vi "FRCts20_Backend_BinarySearchTeamNumber.vi"(8 "error in (no error)":errorcluster) -> (0 "error out":errorcluster)   [LabVIEW 2013, in "FRCts20_Backend_Engine_Deprecated.lvlib"]
doc: "Sorts all teams by team number and performs a binary search through the resulting array of teams. All it does is tell us if the team number was located."
uses:
  FRCts20_Backend_Engine_Deprecated.lvlib
  FRCts20_Backend_TeamDataDfn.ctl
  FRCts20_Backend_TeamDfn.ctl
  FRCts20_Backend_Team_Info.ctl
  FRCts20_Backend_IssueTeamList.ctl
  FRCts20_Backend_IssueDfn.ctl
  FRCts20_Backend_Note_list.ctl
  FRCts20_Backend_Note.ctl
  FRCts20_Backend_request_info.ctl
  FRCts20_Backend_Controls.lvlib
panel:
  out "Found?":bool
  in  "Team Number?":u16
  in  "TeamData":T1
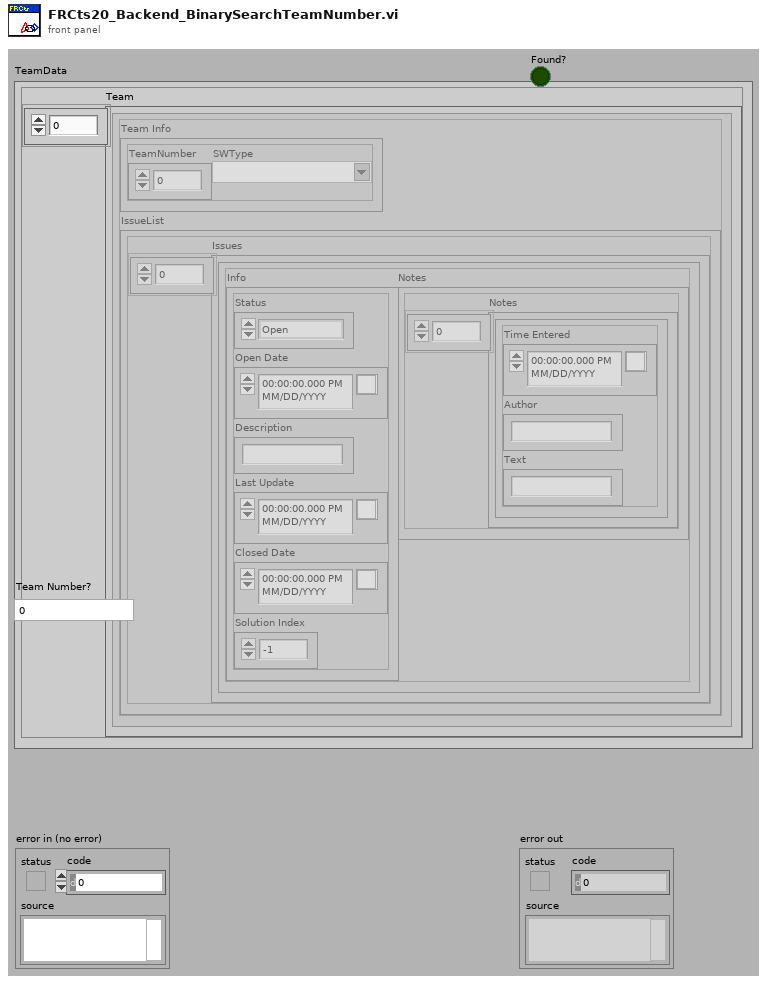
[diagram p1: front panel]
types:
  T1 = typedef "FRCts20_Backend_Controls.lvlib/FRCts20_Backend_TeamDataDfn.ctl" = cluster{"Team":T2[]}
  T2 = typedef "FRCts20_Backend_Controls.lvlib/FRCts20_Backend_TeamDfn.ctl" = cluster{"Team Info":T3, "IssueList":T4}
  T3 = typedef "FRCts20_Backend_Controls.lvlib/FRCts20_Backend_Team_Info.ctl" = cluster{"TeamNumber":u16, "SWType":string}
  T4 = typedef "FRCts20_Backend_Controls.lvlib/FRCts20_Backend_IssueTeamList.ctl" = cluster{"Issues":T5[]}
  T5 = typedef "FRCts20_Backend_Controls.lvlib/FRCts20_Backend_IssueDfn.ctl" = cluster{"Notes":T6, "Info":T8}
  T6 = typedef "FRCts20_Backend_Controls.lvlib/FRCts20_Backend_Note_list.ctl" = cluster{"Notes":T7[]}
  T7 = typedef "FRCts20_Backend_Controls.lvlib/FRCts20_Backend_Note.ctl" = cluster{"Time Entered":timestamp, "Author":string, "Text":string}
  T8 = typedef "FRCts20_Backend_Controls.lvlib/FRCts20_Backend_request_info.ctl" = cluster{"Status":enum16{"Open", "In Work", "Closed"}, "Open Date":timestamp, "Description":string, "Last Update":timestamp, "Closed Date":timestamp, "Solution Index":i32}
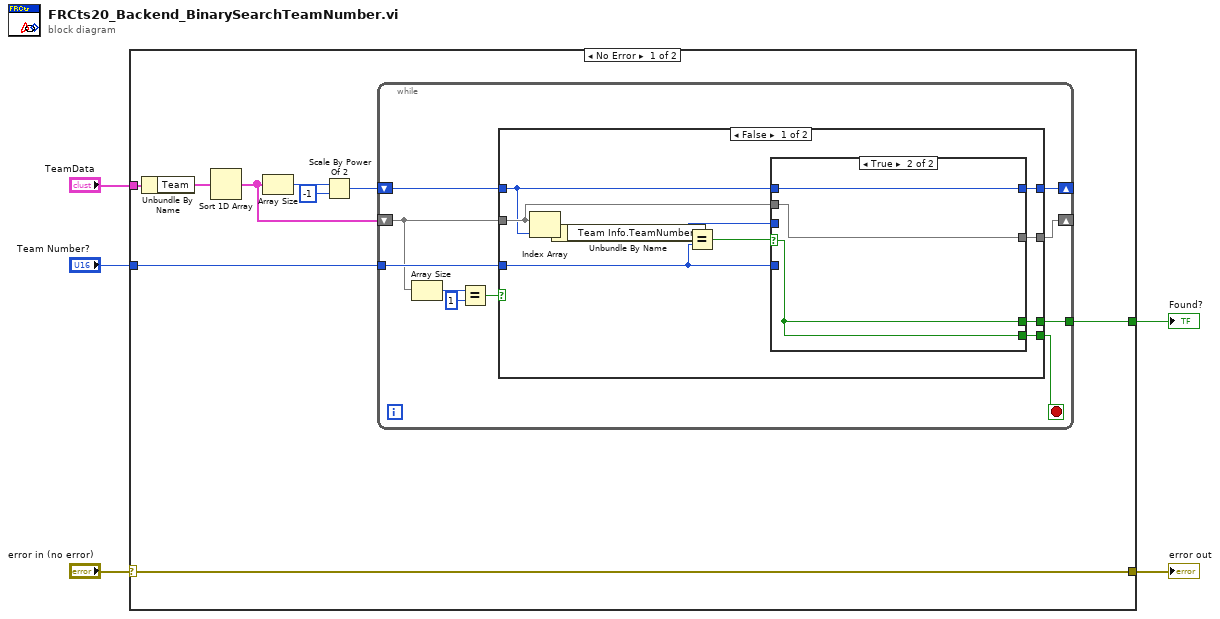
[diagram p0: block diagram]
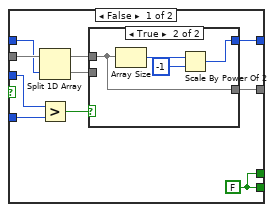
[diagram p2: hidden frame]
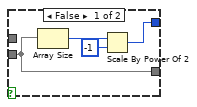
[diagram p3: hidden frame]
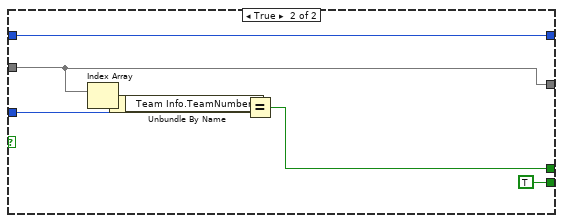
[diagram p4: hidden frame]
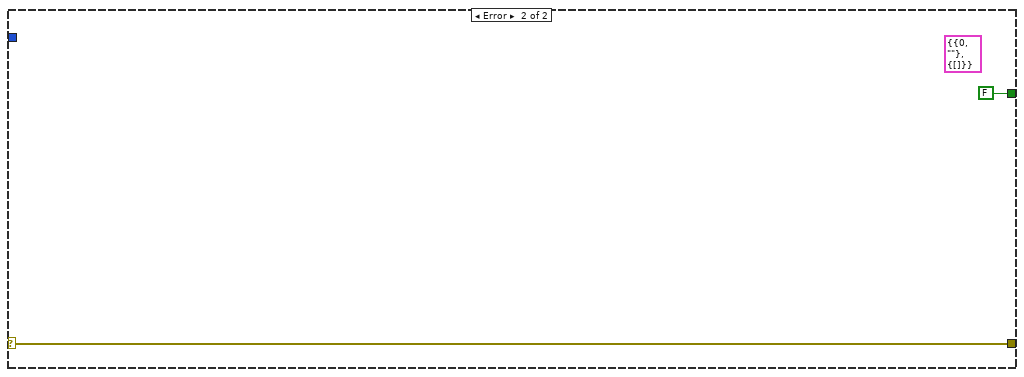
[diagram p5: hidden frame]
diagram:
  n1 = case shown="No Error" "error in (no error)" {
    selector: "error in (no error)" -> [w7 w64]
    tunnel: [w7 w64] -> w4
    tunnel: "TeamData" -> [w14 _]
    tunnel: "Team Number?" -> [w9 _]
    tunnel: [w8 FALSE] -> w1
    frame No Error {
      n2 = Unbundle By Name(w14) -> ("Team"=w13:T2[])
      n3 = Sort 1D Array(array=w13) -> (sorted array=w10:T2[])
      n4 = Array Size(array=w10) -> (size(s)=w12:i32)
      n5 = Scale By Power Of 2(n=w12, x=-1) -> (x*2^n=w6:i32)
      n6 = while {
        tunnel: w9 -> [w24]
        shift-right: [w22] -> _
        shift-left: w6 -> [w17]
        shift-right: [w23] -> _
        shift-left: w10 -> [w20]
        tunnel: [w15] -> w8
        stop <- w21 stop-if-true
        n7 = Array Size(array=w20) -> (size(s)=w19:i32)
        n8 = Equal?(x=w19, y=1) -> (x = y?=w16:bool)
        n9 = case shown="False" w16 {
          tunnel: w24 -> [w32 w61]
          tunnel: [w31 w58] -> w23
          tunnel: [w30 w57] -> w22
          tunnel: [w29 TRUE] -> w21
          tunnel: w20 -> [w28 w58]
          tunnel: w17 -> [w27 w57]
          tunnel: [w26 w60] -> w15
          frame False {
            n10 = Index Array(array=w28, index=w27) -> (element=w25:T2)
            n11 = Unbundle By Name(w25) -> ("Team Info.TeamNumber"=w33:u16)
            n12 = Equal?(x=w33, y=w32) -> (x = y?=w34:bool)
            n13 = case shown="True" w34 {
              selector: w34 -> [_ w55]
              tunnel: [w35 w55] -> w29
              tunnel: w33 -> [w41 _]
              tunnel: w32 -> [w42 _]
              tunnel: w28 -> [w44 w54]
              tunnel: w27 -> [w43 w53]
              tunnel: [w38 w54] -> w31
              tunnel: [w36 w53] -> w30
              tunnel: [w35 w55] -> w26
              frame False {
                w35 = FALSE
                n14 = Split 1D Array(array=w44, index=w43) -> (first subarray=w39:T2[], second subarray=w37:T2[])
                n15 = Greater?(x=w41, y=w42) -> (0:w40:bool)
                n16 = case shown="True" w40 {
                  tunnel: w39 -> [_ w50]
                  tunnel: [w46 w50] -> w38
                  tunnel: w37 -> [w46 _]
                  tunnel: [w45 w49] -> w36
                  frame False {
                    n17 = Array Size(array=w46) -> (size(s)=w47:i32)
                    n18 = Scale By Power Of 2(n=w47, x=-1) -> (x*2^n=w45:i32)
                  }
                  frame True {
                    n19 = Array Size(array=w50) -> (size(s)=w52:i32)
                    n20 = Scale By Power Of 2(n=w52, x=-1) -> (x*2^n=w49:i32)
                  }
                }
              }
              frame True {
              }
            }
          }
          frame True {
            n21 = Index Array(array=w58) -> (element=w56:T2)  [unwired: 1 in]
            n22 = Unbundle By Name(w56) -> ("Team Info.TeamNumber"=w62:u16)
            n23 = Equal?(x=w62, y=w61) -> (x = y?=w60:bool)
          }
        }
      }
    }
    frame Error {
      (unwired) T2 {"Team Info"={"TeamNumber"=0, "SWType"=""}, "IssueList"={"Issues"=[]}} ("Team")
    }
  }
  "error out" <- w4
  "Found?" <- w1
